vi "Open Configuration File.vi"(6 "Configuration File Name":string, 7 "Configuration Directory Path":path, 8 "error in (no error)":errorcluster, 11 "IED in":refnum<class "IED.lvclass">) -> (0 "error out":errorcluster, 2 "config file refnum":T1, 3 "IED out":refnum<class "IED.lvclass">)   [LabVIEW 2015, in "IED Actor.lvlib" / "IED.lvclass"]
doc: "This opens the configuration file and provides a handle to other VIs. If the config file isn't where it's supposed to be this will error."
uses:
  IED.lvclass
  <vilib>/Utility/config.llb/Config Data RefNum.ctl
  <vilib>/Utility/config.llb/NI_LVConfig.lvlib
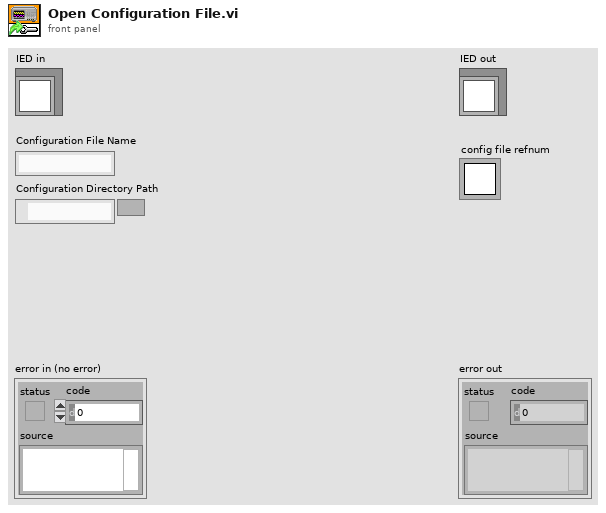
[diagram p1: front panel]
types:
  T1 = typedef "NI_LVConfig.lvlib/Config Data RefNum.ctl" = refnum<k1>
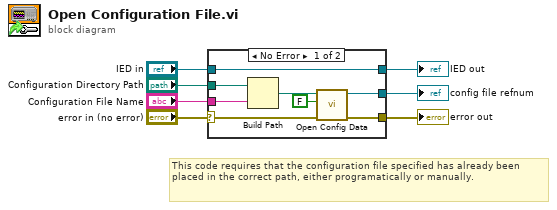
[diagram p0: block diagram]
diagram:
  # "This code requires that the configuration file specified has already been placed in the correct path, either programatically or manually."
  n1 = case shown="No Error" "error in (no error)" {
    selector: "error in (no error)" -> [w13 w17]
    tunnel: [w12 w17] -> w6
    tunnel: [w15 w16] -> w4
    tunnel: "IED in" -> [w15 w16]
    tunnel: "Configuration Directory Path" -> [w11 _]
    tunnel: "Configuration File Name" -> [w10 _]
    tunnel: [w8 _] -> w1
    frame No Error {
      n2 = Build Path(base path=w11, name or relative path=w10) -> (appended path=w9:path)
      n3 = call <vilib>:"Open Config Data.vi"("error in (no error)"=w13, "create file if necessary (T)"=FALSE, "configuration file path"=w9) -> ("error out"=w12:errorcluster, "refnum"=w8:T1)  [unwired: 6 in, 1 out]
    }
    frame Error {
    }
  }
  "error out" <- w6
  "IED out" <- w4
  "config file refnum" <- w1
